vi "Process Data Conifg PID 1 Data line_vel.vi"(11 "출력 클러스터 2":T2) -> (2 "Pos PID gain 1":T1, 3 "Velocity limit 1":cluster{"output high":dbl, "output low":dbl})   [LabVIEW 2019]
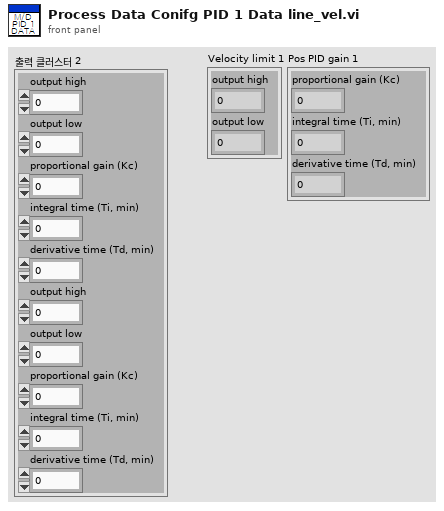
[diagram p1: front panel]
types:
  T1 = cluster{"proportional gain (Kc)":dbl, "integral time (Ti, min)":dbl, "derivative time (Td, min)":dbl}
  T2 = cluster{"output high":dbl, "output low":dbl, "proportional gain (Kc)":dbl, "integral time (Ti, min)":dbl, "derivative time (Td, min)":dbl, "output high":dbl, "output low":dbl, "proportional gain (Kc)":dbl, "integral time (Ti, min)":dbl, "derivative time (Td, min)":dbl}
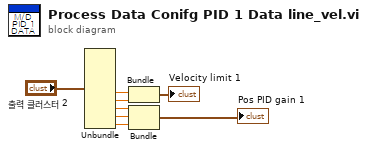
[diagram p0: block diagram]
diagram:
  n1 = Unbundle("출력 클러스터 2") -> ("output high"=w7:dbl, "output low"=w6:dbl, "proportional gain (Kc)"=w5:dbl, "integral time (Ti, min)"=w4:dbl, "derivative time (Td, min)"=w3:dbl)  [unwired: 5 out]
  n2 = Bundle("output high"=w7, "output low"=w6) -> (→"Velocity limit 1":cluster{"output high":dbl, "output low":dbl})  [unwired: 1 in]
  n3 = Bundle("proportional gain (Kc)"=w5, "integral time (Ti, min)"=w4, "derivative time (Td, min)"=w3) -> (→"Pos PID gain 1":T1)  [unwired: 1 in]
